vi "Example.vi"() -> ()   [LabVIEW 2013]
uses:
  <vilib>/NI/Module Execution Interface/Engine Runtime/Execution States.ctl
  <vilib>/NI/Tag Bus Data Framework/Framework Configuration Classes/platypus configuration/class discovery singleton methods.ctl
  Runtime/Standard Engine Runtime.lvclass
  Configuration/Standard Engine Configuration.lvclass
  <vilib>/NI/Module Execution Interface/Engine Runtime/Engine Runtime Interface.lvclass
  <vilib>/NI/Tag Bus Data Framework/Framework Configuration Classes/platypus configuration/PLConfigurationSerializer.lvlib
panel:
  out "State":T1[](array[typedef])
  in  "config. file path":path=path "/home/lvuser/natinst/bin/Web Test.xml"
  out "error out":errorcluster
  in  "stop":bool
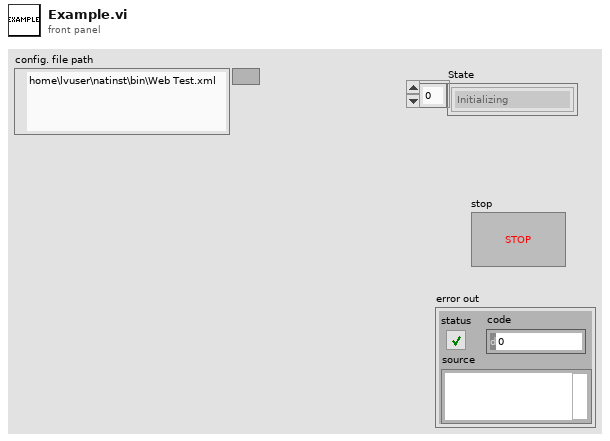
[diagram p1: front panel]
types:
  T1 = typedef "Engine Runtime Interface.lvclass/Execution States.ctl" = enum16{"Initializing", "Paused (Initialized)", "Running", "Set Safe Outputs", "Uninitializing", "Stopped (Uninitialized)", "Error (Uninitialized)", "Safe State (Uninitialized)", "Closed"}
  T2 = typedef "PLConfigurationSerializer.lvlib/class discovery singleton methods.ctl" = enum16{"add search paths", "load class by name"}
  T3 = typedef "PLConfigurationSerializer.lvlib/systems cluster.ctl" = cluster{"System Configuration":refnum<class "PL_System Configuration.lvclass">, "targets":T4[]}
  T4 = typedef "PLConfigurationSerializer.lvlib/targets cluster.ctl" = cluster{"Target Configuration":refnum<class "PL_Target Configuration.lvclass">, "engines":T5[]}
  T5 = typedef "PLConfigurationSerializer.lvlib/engines cluster.ctl" = cluster{"engine configuration":refnum<class "engine configuration.lvclass">, "modules":refnum<class "TBM module configuration.lvclass">[]}
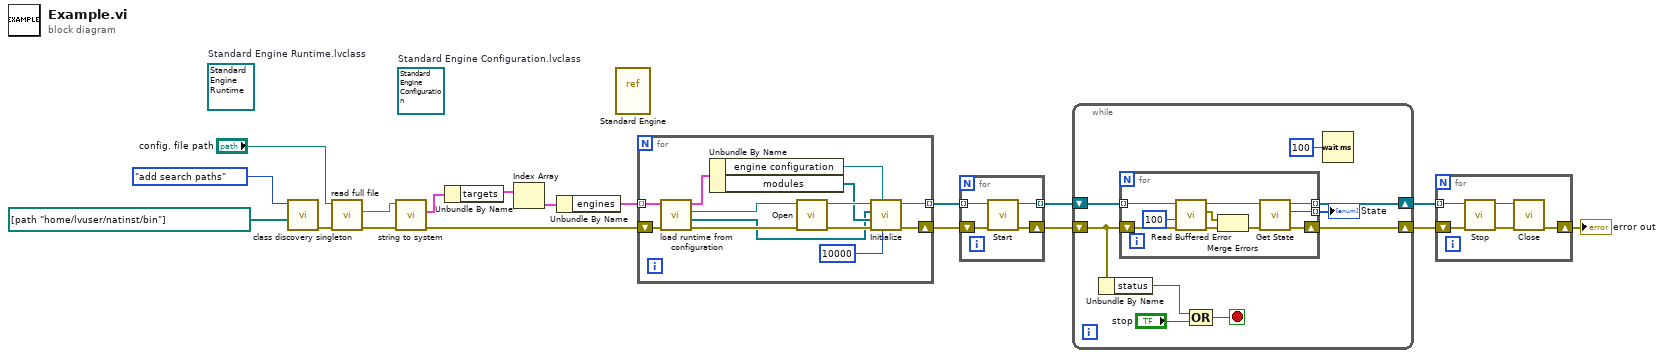
[diagram p0: block diagram]
diagram:
  (unwired) refnum<class "Standard Engine Configuration.lvclass"> refnum  # Standard Engine Configuration.lvclass
  (unwired) refnum<class "Standard Engine Runtime.lvclass"> refnum  # Standard Engine Runtime.lvclass
  n1 = call <vilib>:"class discovery singleton.vi"("Plugin Search Paths"=path[] [path "/home/lvuser/natinst/bin"], "method"=class_discovery_singleton_methods."add search paths") -> ("error out"=w3:errorcluster)  [unwired: 8 in, 1 out]
  n2 = call <vilib>:"read full file.vi"("error in"=w3, "file path"="config. file path") -> ("error out"=w10:errorcluster, "data"=w9:string)  [unwired: 8 in]
  n3 = call <vilib>:"string to system.vi"("error in"=w10, "data"=w9) -> ("error out"=w4:errorcluster, "system"=w8:T3)  [unwired: 8 in]
  n4 = Unbundle By Name(w8) -> ("targets"=w7:T4[])
  n5 = Index Array(array=w7) -> (element=w6:T4)  [unwired: 1 in]
  n6 = Unbundle By Name(w6) -> ("engines"=w5:T5[])
  n7 = vi-ref "Standard Engine.vi"() -> ()  [unwired: 1 out]
  n8 = for {
    tunnel: [w29] -> w18 mode=indexing
    shift-right: [w28] -> w17
    shift-left: w4 -> [w24]
    tunnel: w5 -> [w22] mode=indexing
    n9 = call <vilib>:"load runtime from configuration.vi"("error in"=w24, "engine configuration in"=w22) -> ("error out"=w23:errorcluster, "Component Runtime Objects"=w19:refnum<class "TBM module execution interface.lvclass">[], "Engine Runtime Object"=w20:refnum<class "Engine Runtime Interface.lvclass">, "engine configuration out"=w21:T5)  [unwired: 6 in]
    n10 = Unbundle By Name(w21) -> ("engine configuration"=w26:refnum<class "engine configuration.lvclass">, "modules"=w27:refnum<class "TBM module configuration.lvclass">[])
    n11 = call-dynamic "Open.vi"("error in"=w23, "Engine Runtime Interface in"=w20) -> ("error out"=w30:errorcluster, "Engine Runtime Interface out"=w31:refnum<class "Engine Runtime Interface.lvclass">)  [unwired: 8 in]
    n12 = call-dynamic "Initialize.vi"("timeout in ms"=10000, "Engine Configuration"=w26, "error in"=w30, "module Configurations"=w27, "modules"=w19, "Engine Runtime Interface in"=w31) -> ("error out"=w28:errorcluster, "Engine Runtime Interface out"=w29:refnum<class "Engine Runtime Interface.lvclass">)  [unwired: 4 in]
  }
  n13 = for {
    tunnel: w18 -> [w35] mode=indexing
    tunnel: [w33] -> w13 mode=indexing
    shift-right: [w32] -> w12
    shift-left: w17 -> [w34]
    n14 = call-dynamic "Start.vi"("error in"=w34, "Engine Runtime Interface in"=w35) -> ("error out"=w32:errorcluster, "Engine Runtime Interface out"=w33:refnum<class "Engine Runtime Interface.lvclass">)  [unwired: 8 in]
  }
  n15 = while {
    shift-right: [w39] -> w16
    shift-left: w13 -> [w40]
    shift-right: [w38] -> w15
    shift-left: w12 -> [w36]
    stop <- w41 stop-if-true
    n16 = Unbundle By Name(w36) -> ("status"=w43:bool)
    n17 = for {
      tunnel: w40 -> [w54] mode=indexing
      shift-right: [w48] -> w38
      shift-left: w36 -> [w53]
      tunnel: [w47] -> w39 mode=indexing
      tunnel: [w46] -> w37 mode=indexing
      n18 = call-dynamic "Read Buffered Error.vi"("error in"=w53, "timeout in ms (0)"=100, "Engine Runtime Interface in"=w54) -> ("error out"=w50:errorcluster, "Engine Error"=w51:errorcluster, "Engine Runtime Interface out"=w52:refnum<class "Engine Runtime Interface.lvclass">)  [unwired: 6 in]
      n19 = Merge Errors(w51, w50) -> (w49:errorcluster)
      n20 = call-dynamic "Get State.vi"("error in"=w49, "Engine Runtime Interface in"=w52) -> ("error out"=w48:errorcluster, "Engine State"=w46:T1, "Engine Runtime Interface out"=w47:refnum<class "Engine Runtime Interface.lvclass">)  [unwired: 7 in]
    }
    "State" <- w37
    n21 = Compound Arithmetic op=OR(w43, "stop") -> (w41:bool)
    n22 = Wait (ms)(milliseconds to wait=u32 100) -> ()  [unwired: 1 out]
  }
  n23 = for {
    tunnel: w16 -> [w57] mode=indexing
    shift-right: [w55] -> w14
    shift-left: w15 -> [w56]
    n24 = call-dynamic "Stop.vi"("error in"=w56, "Engine Runtime Interface in"=w57) -> ("error out"=w58:errorcluster, "Engine Runtime Interface out"=w59:refnum<class "Engine Runtime Interface.lvclass">)  [unwired: 8 in]
    n25 = call-dynamic "Close.vi"("error in"=w58, "Engine Runtime Interface in"=w59) -> ("error out"=w55:errorcluster)  [unwired: 9 in]
  }
  "error out" <- w14
